vi "Get Table Configuration.vi"(8 "error in (no error)":errorcluster, 11 "Form from Configured Table in":refnum<class "Form from Configured Table.lvclass">) -> (0 "error out":errorcluster, 2 "Table Configuration":refnum<class "Table Configuration Interface.lvclass">, 3 "Form from Configured Table out":refnum<class "Form from Configured Table.lvclass">)   [LabVIEW 2020]
uses:
  Database OOP/Table Libraries/Table Configuration Interface/Table Configuration Interface.lvclass
  Form from Configured Table.lvclass
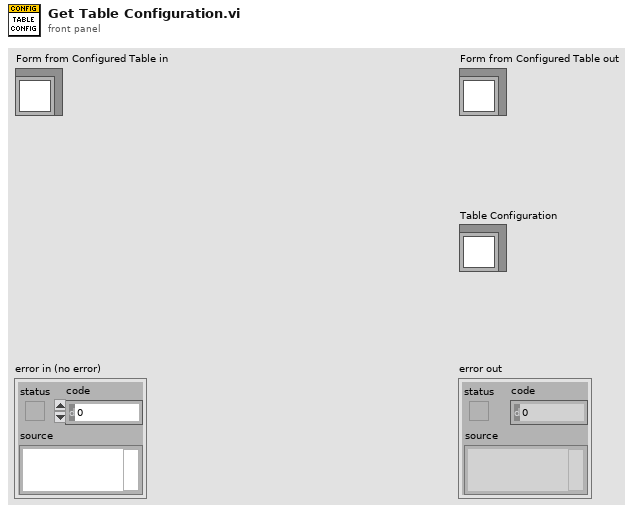
[diagram p1: front panel]
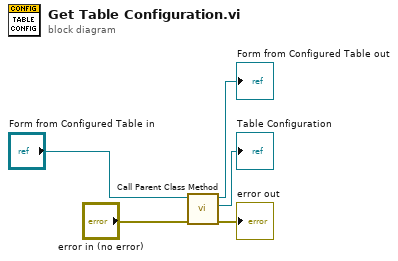
[diagram p0: block diagram]
diagram:
  n1 = call-parent "Call Parent Class Method"("error in (no error)"="error in (no error)", "Panel Form Controller Configuration in"="Form from Configured Table in") -> ("error out"=→"error out":errorcluster, "Table Configuration"=→"Table Configuration":refnum<class "Table Configuration Interface.lvclass">, "Panel Form Controller Configuration out"=→"Form from Configured Table out":refnum<class "Form from Configured Table.lvclass">)  [unwired: 7 in]
